vi "Focus Found Estimation.vi"() -> ()   [LabVIEW 2014]
panel:
  in  "Top Range":i32=10
  out "XY Graph":cluster{i32[], sgl[]}[](graph)
  in  "Matching Curves":cluster{"Z":dbl[], "Score":sgl[]}[](array[cluster])
  # "LICENSED MATERIALS – PROPERTY OF IBM\nCopyright IBM Corp. 2016, 2016\nALL RIGHTS RESERVED"
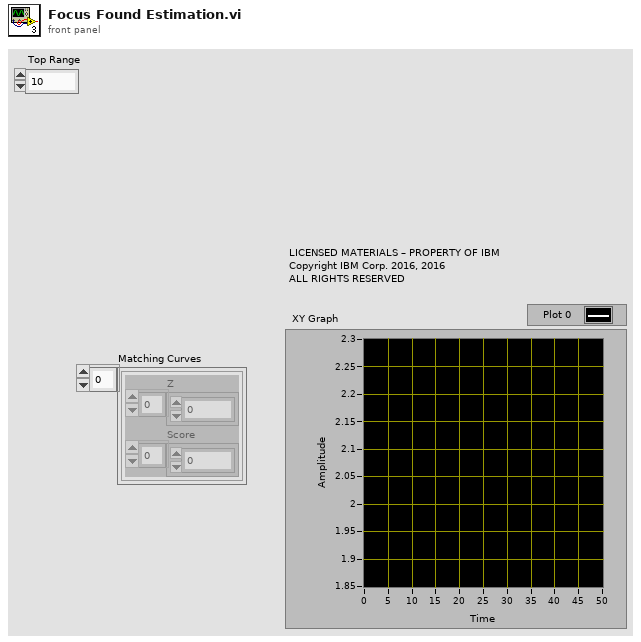
[diagram p1: front panel]
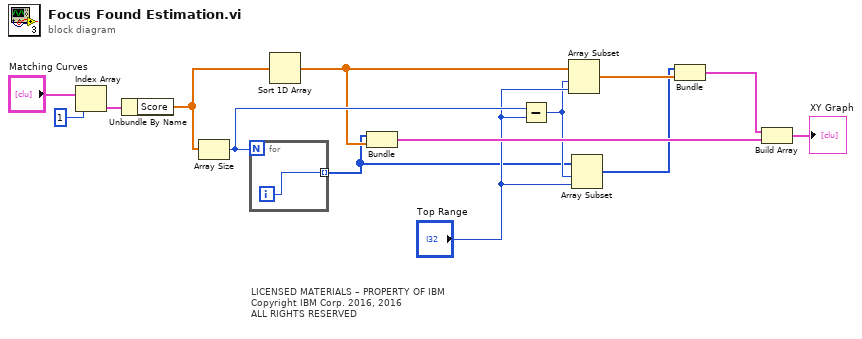
[diagram p0: block diagram]
diagram:
  # "LICENSED MATERIALS – PROPERTY OF IBM\nCopyright IBM Corp. 2016, 2016\nALL RIGHTS RESERVED"
  n1 = Index Array(array="Matching Curves", index=1) -> (element=w12:cluster{"Z":dbl[], "Score":sgl[]})
  n2 = Unbundle By Name(w12) -> ("Score"=w11:sgl[])
  n3 = Array Size(array=w11) -> (size(s)=w9:i32)
  n4 = for {
    N: w9 -> [_]
    tunnel: [w15] -> w3 mode=indexing
    i -> [w15]
  }
  n5 = Sort 1D Array(array=w11) -> (sorted array=w6:sgl[])
  n6 = Bundle(w3, w6) -> (w10:cluster{i32[], sgl[]})  [unwired: 1 in]
  n7 = Subtract(x=w9, y="Top Range") -> (x-y=w4:i32)
  n8 = Array Subset(array=w6, index=w4, length="Top Range") -> (w8:sgl[])
  n9 = Array Subset(array=w3, index=w4, length="Top Range") -> (w2:i32[])
  n10 = Bundle(w2, w8) -> (w1:cluster{i32[], sgl[]})  [unwired: 1 in]
  n11 = Build Array(w1, w10) -> (→"XY Graph":cluster{i32[], sgl[]}[])
